vi "Generate Rd Cmd.vi"(1 "Number of Elements":u32=8388608 format="%.0x", 7 "next Read request":T1, 11 "Ready for Read":bool) -> (4 "ready for input":bool, 6 "Address":u32, 15 "Valid?":bool)   [LabVIEW 2013]
uses:
  Read Request Command.ctl
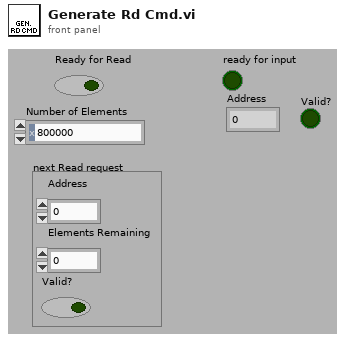
[diagram p1: front panel]
types:
  T1 = typedef "Read Request Command.ctl" = cluster{"Address":u32, "Elements Remaining":u32, "Valid?":bool}
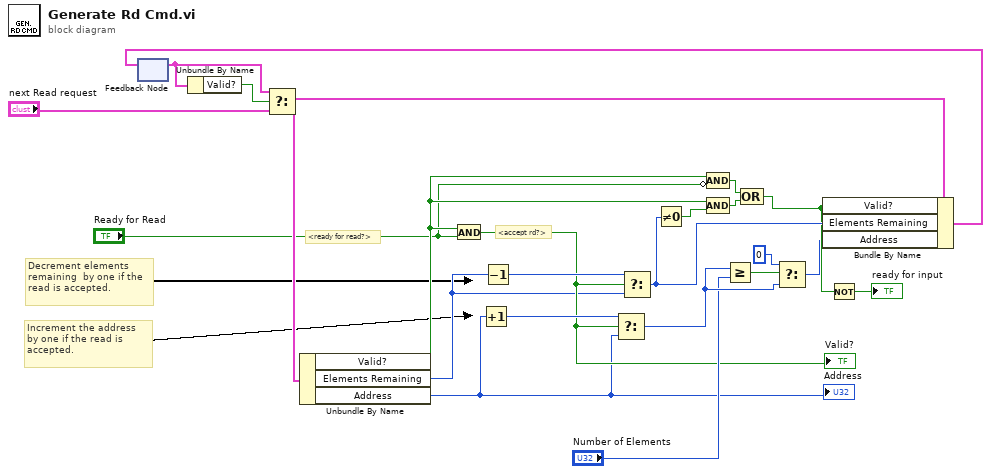
[diagram p0: block diagram]
diagram:
  # "Increment the address  by one if the read is accepted."
  # "Decrement elements remaining  by one if the read is accepted."
  # "<ready for read?>"
  # "<accept rd?>"
  n1 = feedback #1() -> (w21:T1)  [unwired: 1 in]
  n2 = Unbundle By Name(w21) -> ("Valid?"=w22:bool)
  n3 = Select(t=w21, s=w22, f="next Read request") -> (s? t:f=w19:T1)
  n4 = Unbundle By Name(w19) -> ("Valid?"=w12:bool, "Elements Remaining"=w2:u32, "Address"=w1:u32)
  "Address" <- w1
  n5 = And(x=w12, y="Ready for Read") -> (x .and. y?=w4:bool)
  "Valid?" <- w4
  n6 = Increment(x=w1) -> (x+1=w10:u32)
  n7 = Decrement(x=w2) -> (x-1=w18:u32)
  n8 = Select(t=w10, s=w4, f=w1) -> (s? t:f=w8:u32)
  n9 = Select(t=w18, s=w4, f=w2) -> (s? t:f=w17:u32)
  n10 = Not Equal To 0?(x=w17) -> (x != 0?=w16:bool)
  n11 = Compound Arithmetic op=AND(w12, invert "Ready for Read") -> (w14:bool)
  n12 = Compound Arithmetic op=AND(w12, w16) -> (w15:bool)
  n13 = Greater Or Equal?(x=w8, y="Number of Elements") -> (x >= y?=w9:bool)
  n14 = Compound Arithmetic op=OR(w14, w15) -> (w11:bool)
  n15 = Select(t=u32 0, s=w9, f=w8) -> (s? t:f=w5:u32)
  n16 = Bundle By Name(cluster=w19, "Valid?"=w11, "Elements Remaining"=w17, "Address"=w5) -> (w20:T1)
  n17 = feedback-in #1(w20) -> ()
  n18 = Not(x=w11) -> (.not. x?=→"ready for input":bool)
